vi "Configure TS Panel.vi"(8 "error in":errorcluster, 11 "Test Stand in":refnum<class "Cryo Sep Test Stand.lvclass">) -> (0 "error out":errorcluster, 3 "Test Stand out":refnum<class "Cryo Sep Test Stand.lvclass">)   [LabVIEW 2019, in "Test Stands.lvlib" / "Cryo Sep Test Stand.lvclass"]
uses:
  Cryo Sep Test Stand.lvclass
  Results/Cryo Sep Results/Cryo Sep Front Panel.vi
  Generic Test Stand/Generic Test Stand.lvclass
  C:/Users/wg/Documents/LV_Projects/test-stand/App/Generic Test Stand/Generic Test Stand.lvclass
  Results/Cryo Sep Results/Cryo Sep Results.lvclass
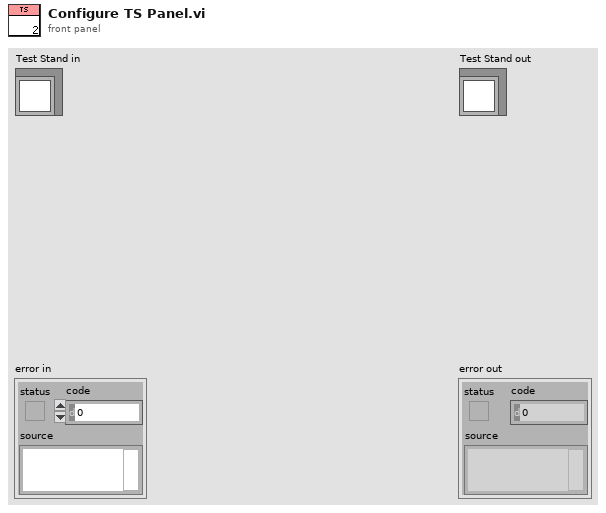
[diagram p1: front panel]
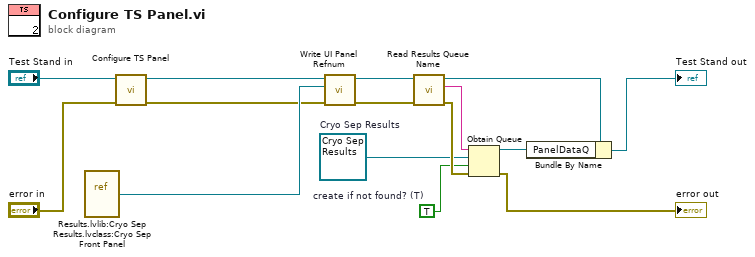
[diagram p0: block diagram]
diagram:
  w2 = refnum<class "Cryo Sep Results.lvclass"> refnum  # Cryo Sep Results
  w4 = TRUE  # create if not found? (T)
  n1 = vi-ref "Results.lvlib:Cryo Sep Results.lvclass:Cryo Sep Front Panel.vi"() -> (w15:refnum<vi>)
  n2 = call-parent "Configure TS Panel.vi"("error in (no error)"="error in", "Generic Test Stand in"="Test Stand in") -> ("error out"=w11:errorcluster, "Generic Test Stand out"=w13:refnum<class "Cryo Sep Test Stand.lvclass">)  [unwired: 8 in]
  n3 = call "Write UI Panel Refnum.vi"("error in (no error)"=w11, "UI Panel Refnum"=w15, "Generic Test Stand in"=w13) -> ("error out"=w7:errorcluster, "Generic Test Stand out"=w10:refnum<class "Cryo Sep Test Stand.lvclass">)  [unwired: 7 in]
  n4 = call "Read Results Queue Name.vi"("error in (no error)"=w7, "Generic Test Stand in"=w10) -> ("error out"=w5:errorcluster, "Results Queue Name"=w6:string, "Generic Test Stand out"=w9:refnum<class "Cryo Sep Test Stand.lvclass">)  [unwired: 7 in]
  n5 = Obtain Queue(name (unnamed)=w6, element data type=w2, create if not found? (T)=w4, error in (no error)=w5) -> (queue out=w1:refnum<queue>, error out=→"error out":errorcluster)  [unwired: 1 in, 1 out]
  n6 = Bundle By Name(cluster=w9, "PanelDataQ"=w1) -> (→"Test Stand out":refnum<class "Cryo Sep Test Stand.lvclass">)
